vi "senddata.vi"(0 "object in":refnum<class "interface.lvclass">, 1 "发送报文":string, 5 "error in (no error)":errorcluster) -> (14 "object out":refnum<class "interface.lvclass">, 19 "error out":errorcluster)   [LabVIEW 2016, in "interface.lvclass"]
uses:
  interface.lvclass
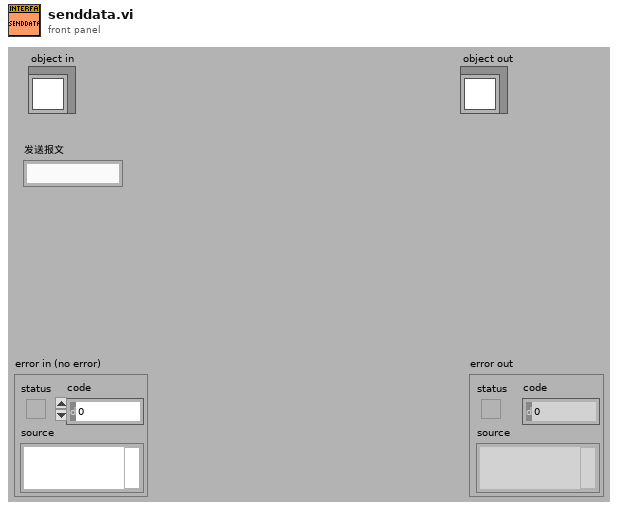
[diagram p1: front panel]
types:
  T1 = cluster{"枚举":enum16{"打开连接", "发送数据", "读取数据", "数据处理", "关闭连接"}, "发送报文":string}
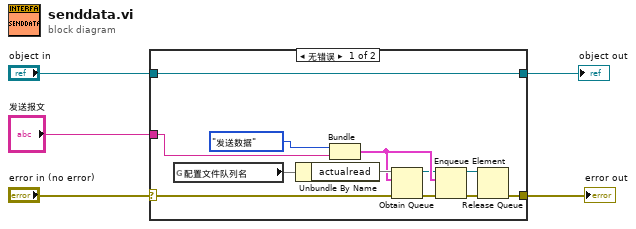
[diagram p0: block diagram]
diagram:
  n1 = case shown="无错误" "error in (no error)" {
    selector: "error in (no error)" -> [w7 w19]
    tunnel: [w6 w19] -> w4
    tunnel: [w8 w18] -> w2
    tunnel: "object in" -> [w8 w18]
    tunnel: "发送报文" -> [w12 _]
    frame No Error {
      n2 = global read "断电保存全局.vi" "配置文件队列名"() -> (w17)
      n3 = Unbundle By Name(w17) -> ("actualread"=w14)
      n4 = Bundle("枚举"=enum16{"打开连接", "发送数据", "读取数据", "数据处理", "关闭连接"}."发送数据", "发送报文"=w12) -> (w11:T1)  [unwired: 1 in]
      n5 = Obtain Queue(name (unnamed)=w14, element data type=w11, error in (no error)=w7) -> (queue out=w10:refnum<queue>, error out=w9:errorcluster)  [unwired: 2 in, 1 out]
      n6 = Enqueue Element(queue=w10, element=w11, error in (no error)=w9) -> (queue out=w16:refnum<queue>, error out=w15:errorcluster)  [unwired: 1 in, 1 out]
      n7 = Release Queue(queue=w16, error in (no error)=w15) -> (error out=w6:errorcluster)  [unwired: 1 in, 2 out]
    }
    frame Error {
    }
  }
  "error out" <- w4
  "object out" <- w2
